vi "Align Panel Objects.vi"(8 "error in (no error)":errorcluster, 10 "Align Type":T1, 11 "Panel Objects in":refnum<class "Panel Object.lvclass">[](array[class])) -> (0 "error out":errorcluster, 3 "Panel Objects out":refnum<class "Panel Object.lvclass">[](array[class]))   [LabVIEW 2018, in "Panel Object.lvclass"]
uses:
  <resource>/dialog/QuickDrop/plugins/PaneRelief/Classes/Panel Object/Panel Object.lvclass
  <resource>/dialog/QuickDrop/plugins/PaneRelief/Classes/Panel Object/Align Type--Enum.ctl
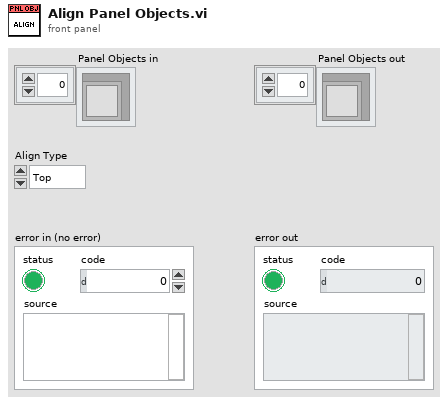
[diagram p1: front panel]
types:
  T1 = typedef "Align Type--Enum.ctl" = enum16{"Top", "Bottom", "Left", "Right"}
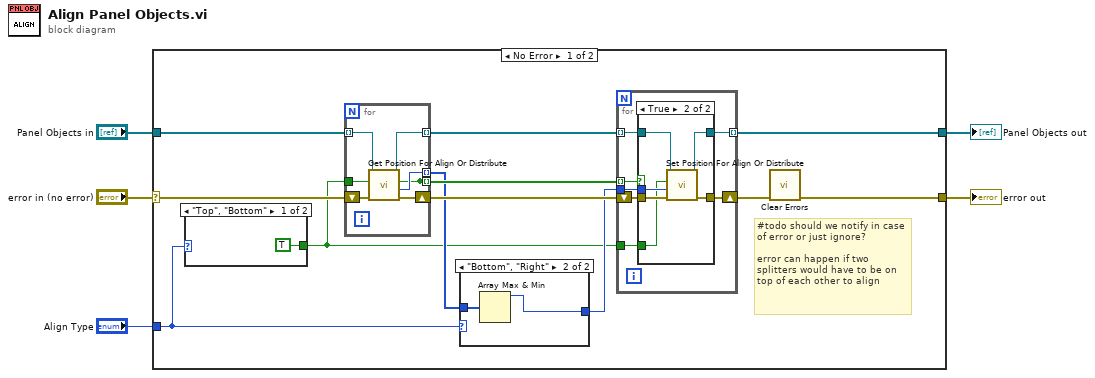
[diagram p0: block diagram]
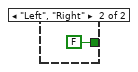
[diagram p2: hidden frame]
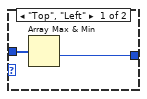
[diagram p3: hidden frame]
diagram:
  n1 = case shown="No Error" "error in (no error)" {
    selector: "error in (no error)" -> [w9 w46]
    tunnel: [w16 w47] -> w5
    tunnel: "Panel Objects in" -> [w10 w47]
    tunnel: [w8 w46] -> w2
    tunnel: "Align Type" -> [w6 _]
    frame No Error {
      # "#todo should we notify in case of error or just ignore?\n\nerror can happen if two splitters would have to be on top of each other to align"
      n2 = case shown="\"Top\", \"Bottom\"" w6 {
        tunnel: [TRUE FALSE] -> w7
        frame "Top", "Bottom" {
        }
        frame "Left", "Right" {
        }
      }
      n3 = for {
        shift-right: [w42] -> w13
        shift-left: w9 -> [w45]
        tunnel: w10 -> [w44] mode=indexing
        tunnel: [w43] -> w15 mode=indexing
        tunnel: [w41] -> w11 mode=indexing if=w40
        tunnel: [w40] -> w17 mode=indexing
        tunnel: w7 -> [w39]
        n4 = call-dynamic "Get Position For Align Or Distribute.vi"("Error In"=w45, "Vertical? (F: Horizontal)"=w39, "Panel Object in"=w44) -> ("Error Out"=w42:errorcluster, "Position"=w41:i32, "Applicable?"=w40:bool, "Panel Object out"=w43:refnum<class "Panel Object.lvclass">)  [unwired: 5 in]
      }
      n5 = case shown="\"Bottom\", \"Right\"" w6 {
        tunnel: [w20 w22] -> w12
        tunnel: w11 -> [w21 w23]
        frame "Top", "Left" {
          n6 = Array Max & Min(array=w21) -> (min value=w20:i32)  [unwired: 3 out]
        }
        frame "Bottom", "Right" {
          n7 = Array Max & Min(array=w23) -> (max value=w22:i32)  [unwired: 3 out]
        }
      }
      n8 = for {
        tunnel: w12 -> [w30]
        shift-right: [w28] -> w14
        shift-left: w13 -> [w29]
        tunnel: w15 -> [w27] mode=indexing
        tunnel: [w26] -> w16 mode=indexing
        tunnel: w17 -> [w25] mode=indexing
        tunnel: w7 -> [w24]
        n9 = case shown="True" w25 {
          tunnel: w30 -> [_ w38]
          tunnel: w29 -> [w31 w37]
          tunnel: [w31 w36] -> w28
          tunnel: w27 -> [w32 w35]
          tunnel: [w32 w34] -> w26
          tunnel: w24 -> [_ w33]
          frame False {
          }
          frame True {
            n10 = call-dynamic "Set Position For Align Or Distribute.vi"("Error In"=w37, "Position"=w38, "Vertical? (F: Horizontal)"=w33, "Panel Object in"=w35) -> ("Error Out"=w36:errorcluster, "Panel Object out"=w34:refnum<class "Panel Object.lvclass">)  [unwired: 6 in]
          }
        }
      }
      n11 = call <vilib>:"Clear Errors.vi"("error in (no error)"=w14) -> ("error out"=w8:errorcluster)  [unwired: 5 in, 1 out]
    }
    frame Error {
    }
  }
  "Panel Objects out" <- w5
  "error out" <- w2
